vi "IntegrationTime-global.vi"() -> ()   [LabVIEW 2013]
panel:
  out "Time Constant (8: 100ms) 2":u16(ring)=8 items=["10 us", "30 us", "100 us", "300 us", "1 ms", "3 ms", "10 ms", "30 ms", "100 ms", "300 ms", "1 s", "3 s", "10 s", "30 s", "100 s", "300 s", "1 ks", "3 ks", "10 ks", "30 ks"]
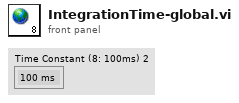
[diagram p1: front panel]
diagram:
